vi "stopCaptureImage.vi"(8 "error in (no error)":errorcluster, 9 "command_stopImageCapture":T1, 10 "CommandID":i32, 11 "ContextThisComponent in":refnum<class "ContextThisComponent.lvclass">) -> (0 "error out":errorcluster, 3 "ContextThisComponent out":refnum<class "ContextThisComponent.lvclass">)   [LabVIEW 2016, in "ContextThisComponent.lvclass"]
uses:
  ContextThisComponent.lvclass
  ts_sallv_sedspectrometer/DataTypes/command_stopImageCapture.ctl
  ContextThisComponent.lvclass/ContextThisComponent.ctl
  IStateFactory/IStateFactory.lvclass
  IModel/IModel.lvclass
  State/State.lvclass
  ts_sallv_sedspectrometer/SALLV_sedSpectrometer.lvlib
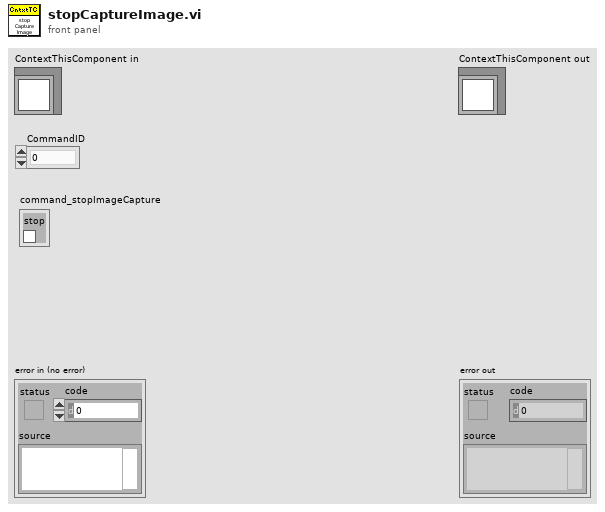
[diagram p1: front panel]
types:
  T1 = typedef "SALLV_sedSpectrometer.lvlib/command_stopImageCapture.ctl" = cluster{"stop":bool}
  T2 = typedef "SALLV_sedSpectrometer.lvlib/logevent_DetailedState.ctl" = cluster{"detailedState":enum32{"", "DisabledState", "EnabledState", "FaultState", "OfflineState", "StandbyState", "CaptureSpectImage", "NotImaging"}, "priority":i32}
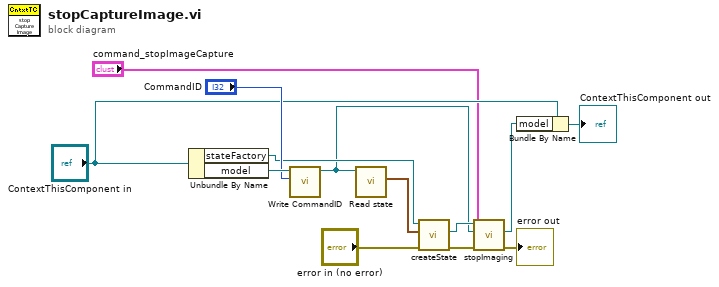
[diagram p0: block diagram]
diagram:
  n1 = Unbundle By Name("ContextThisComponent in") -> ("stateFactory"=w11:refnum<class "IStateFactory.lvclass">, "model"=w13:refnum<class "IModel.lvclass">)
  n2 = call-dynamic "Write CommandID.vi"("CommandID"="CommandID", "IModel in"=w13) -> ("IModel out"=w7:refnum<class "IModel.lvclass">)  [unwired: 8 in, 1 out]
  n3 = call-dynamic "Read state.vi"("IModel in"=w7) -> ("DetailedState"=w10:T2)  [unwired: 9 in, 1 out]
  n4 = call-dynamic "createState.vi"("error in (no error)"="error in (no error)", "DetailedState"=w10, "IStateFactory in"=w11) -> ("error out"=w6:errorcluster, "state"=w8:refnum<class "State.lvclass">)  [unwired: 6 in, 1 out]
  n5 = call-dynamic "stopImaging.vi"("error in (no error)"=w6, "command_stopImageCapture"="command_stopImageCapture", "model in"=w7, "State in"=w8) -> ("error out"=→"error out":errorcluster, "model out"=w2:refnum<class "IModel.lvclass">)  [unwired: 5 in, 1 out]
  n6 = Bundle By Name(cluster="ContextThisComponent in", "model"=w2) -> (→"ContextThisComponent out":refnum<class "ContextThisComponent.lvclass">)
